vi "FilterBatteryVoltage.vi"(10 "NotifierReff 2":T1, 11 "Queue in":refnum<queue>) -> ()   [LabVIEW 2013]
uses:
  Data/TypeDefs/Notifiers.ctl
  Data/TypeDefs/UTM Location.ctl
  Data/TypeDefs/GPS Sensor Status.ctl
  Data/TypeDefs/Sail Set Suggestions.ctl
  Data/TypeDefs/Rudder Set Suggestions.ctl
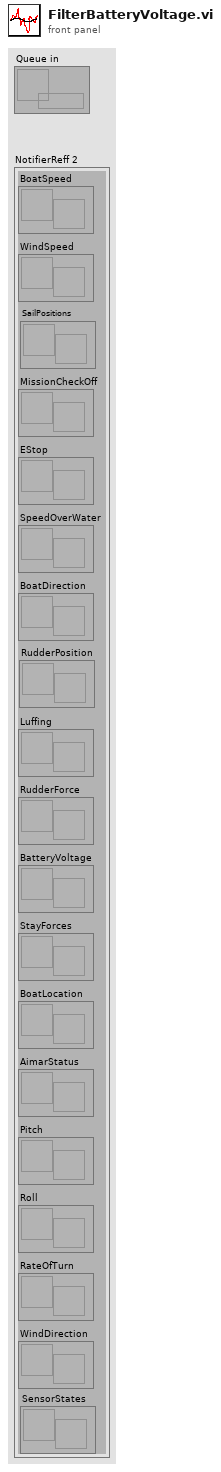
[diagram p1: front panel]
types:
  T1 = typedef "Notifiers.ctl" = cluster{"BoatSpeed":refnum<notifier>, "WindSpeed":refnum<notifier>, "MissionCheckOff":refnum<notifier>, "EStop":refnum<notifier>, "SpeedOverWater":refnum<notifier>, "BoatDirection":refnum<notifier>, "Luffing":refnum<notifier>, "RudderForce":refnum<notifier>, "BatteryVoltage":refnum<notifier>, "StayForces":refnum<notifier>, "BoatLocation":refnum<notifier>, "AimarStatus":refnum<notifier>, "Pitch":refnum<notifier>, "Roll":refnum<notifier>, "RateOfTurn":refnum<notifier>, "WindDirection":refnum<notifier>, "SailPositions":refnum<notifier>, "RudderPosition":refnum<notifier>, "SensorStates":refnum<notifier>}
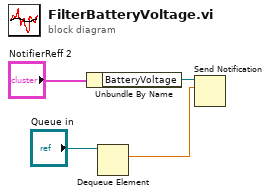
[diagram p0: block diagram]
diagram:
  n1 = Unbundle By Name("NotifierReff 2") -> ("BatteryVoltage"=w1:refnum<notifier>)
  n2 = Dequeue Element(queue="Queue in") -> (element=w4:dbl)  [unwired: 2 in, 3 out]
  n3 = Send Notification(notification=w4, notifier=w1) -> ()  [unwired: 1 in, 2 out]
